vi "Loop_SM.vi"() -> ()   [LabVIEW 2017, in "Lift.lvlib"]
uses:
  Lift.lvlib
  CLUSTER_CMD_SM_Lift_Rotate.ctl
  ENUM_SM_Rotate_Positions.ctl
  _SHARE ALL/TypeDef Share All/CLUSTER_TalonInput.ctl
  System Drivers/Phoenix-LabVIEW/Motor Controller/Controls/CTRE_Phoenix_MotorControl_ControlMode.ctl
  TypeDef/CLUSTER_PID.ctl
  ENUM_SM_State.ctl
  CLUSTER_ACT_Lift Output.ctl
  _SHARE ALL/RoboRio Share All/SRX Share All/TypeDefs SRX/Cluster_SRX_General Data.ctl
  _SHARE ALL/RoboRio Share All/SRX Share All/TypeDefs SRX/Cluster_SRX_Common Runtime Data.ctl
  _SHARE ALL/RoboRio Share All/SRX Share All/TypeDefs SRX/Cluster_SRX_Error Calculations.ctl
  _SHARE ALL/RoboRio Share All/SRX Share All/TypeDefs SRX/Cluster_SRX_Voltage Out Data.ctl
  _SHARE ALL/RoboRio Share All/SRX Share All/TypeDefs SRX/Cluster_SRX_Sensor Out Data.ctl
  _SHARE ALL/RoboRio Share All/SRX Share All/TypeDefs SRX/Cluster_SRX_Sensor Quad Data.ctl
  _SHARE ALL/RoboRio Share All/SRX Share All/TypeDefs SRX/Cluster_SRX_Analog In Data.ctl
  _SHARE ALL/RoboRio Share All/SRX Share All/TypeDefs SRX/Cluster_SRX_PWM Sensor Data.ctl
  _SHARE ALL/RoboRio Share All/SRX Share All/TypeDefs SRX/Cluster_SRX_F and R Limit Indicators.ctl
  ENUM_SM_Action.ctl
  Globals/Global_Device_IDs.vi
  _SHARE ALL/Global Share All/Global_STOP.vi
  Global_CMD.vi
  Global_ACT Write_Data Out.vi
  Global_SM Write_Data Out.vi
panel:
  out "State":T1
  out "SM Output":T2 {"Talon Mode" items=["PercentOutput"=0, "Position"=1, "Velocity"=2, "Current"=3, "Follower"=5, "MotionProfile"=6, "MotionMagic"=7, "MotionMagicArc"=8, "MotionProfileArc"=10, "Disabled"=15]}
  out "SM CMD Input":T5={"Enable System"=TRUE, "Rotate Position"=enum."Neutral: 0", "Manual Velocity"=0.0, "Manual Mode"=FALSE}
  out "Cycle Time (S)":dbl format="%.3g"
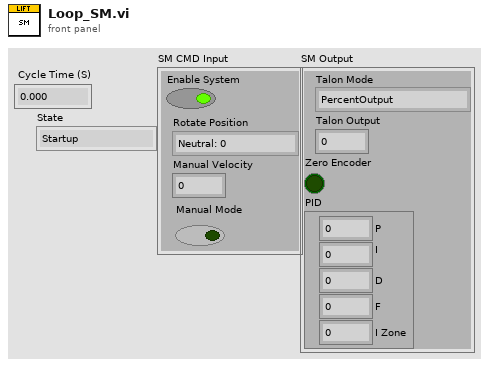
[diagram p1: front panel]
types:
  T1 = typedef "Lift.lvlib/ENUM_SM_State.ctl" = enum16{"Startup", "Idle", "Manual", "Position - Moving", "Position - Holding", "Shutdown"}
  T2 = typedef "CLUSTER_TalonInput.ctl" = cluster{"Talon Mode":T3, "Talon Output":dbl, "Zero Encoder":bool, "PID":T4}
  T3 = typedef "CTRE_Phoenix_MotorControl_ControlMode.ctl" = u16
  T4 = typedef "CLUSTER_PID.ctl" = cluster{"P":dbl, "I":dbl, "D":dbl, "F":dbl, "I Zone":dbl}
  T5 = typedef "Lift.lvlib/CLUSTER_CMD_SM_Lift_Rotate.ctl" = cluster{"Enable System":bool, "Rotate Position":T6, "Manual Velocity":dbl, "Manual Mode":bool}
  T6 = typedef "Lift.lvlib/ENUM_SM_Rotate_Positions.ctl" = enum16{"Neutral: 0", "Pickup: 0", "Exchange: 0", "Switch: 0", "Scale: 0", "Climb: 0"}
  T7 = typedef "Lift.lvlib/CLUSTER_ACT_Lift Output.ctl" = cluster{"Device Info Out":T8, "Common Runtime Data Out":T9, "Quad Sensor Data Out":T13, "Analog Sensor Data Out":T14, "PWM Data Out":T15, "Hard Limits Out":T16}
  T8 = typedef "Cluster_SRX_General Data.ctl" = cluster{"Device ID":i32, "Firmware Version":i32, "Inverted?":bool, "Has Reset Occurred?":bool}
  T9 = typedef "Cluster_SRX_Common Runtime Data.ctl" = cluster{"Calc":T10, "Voltage ":T11, "Sensor":T12, "Current":dbl, "Temp":dbl}
  T10 = typedef "Cluster_SRX_Error Calculations.ctl" = cluster{"Error":i32, "D-Error":dbl, "I-Acc":dbl}
  T11 = typedef "Cluster_SRX_Voltage Out Data.ctl" = cluster{"Percent":dbl, "Output":dbl, "Bus":dbl}
  T12 = typedef "Cluster_SRX_Sensor Out Data.ctl" = cluster{"Pos":i32, "Vel":i32}
  T13 = typedef "Cluster_SRX_Sensor Quad Data.ctl" = cluster{"Position":i32, "Velocity":i32, "Quad A Pin":bool, "Quad B Pin":bool, "Quad Idx Pin":bool}
  T14 = typedef "Cluster_SRX_Analog In Data.ctl" = cluster{"WithOv":i32, "Raw":i32, "Velocity":i32}
  T15 = typedef "Cluster_SRX_PWM Sensor Data.ctl" = cluster{"Position":i32, "Velocity":i32, "High(us)":i32, "Period(us)":i32}
  T16 = typedef "Cluster_SRX_F and R Limit Indicators.ctl" = cluster{"Forward Closed?":bool, "Reverse Closed?":bool}
  T17 = typedef "Lift.lvlib/ENUM_SM_Action.ctl" = enum16{"No Action", "Reset Time", "Reset All", "Reset Encoder", "Manual", "Position", "Set PID 1", "Disable Motor"}
  T18 = typedef "CLUSTER_Arm_Device_IDs.ctl" = cluster{"Master":T19, "Slave":T19}
  T19 = typedef "CLUSTER_Talon_Setup.ctl" = cluster{"Open Data":T20, "Current Config Data":T21, "Sensor Config":T22, "Hard Limits":T24, "Motion Magic Config Data":T26, "PIDF":T27, "Maximum Integral Accumulator Value":dbl, "AllowableClosedLoop":i32, "Limits":T28, "Output Config":T29}
  T20 = typedef "Cluster_SRX_OPEN Data.ctl" = cluster{"SRX ID":u8, "Invert Output":bool}
  T21 = typedef "Cluster_SRX_Current Config.ctl" = cluster{"Enable Current Limit?":bool, "Peak Current (Amps)":i32, "Peak Current Maximum Duration (ms)":i32, "Continuous Current Limit (Amps)":i32}
  T22 = typedef "Cluster_SRX_Sensor Config.ctl" = cluster{"Feedback Device":T23, "PhaseSensor":bool}
  T23 = typedef "CTRE_Phoenix_MotorControl_FeedbackDevice.ctl" = i8
  T24 = typedef "Cluster_SRX_Config Hard Limits.ctl" = cluster{"Fwd Enable":bool, "Rev Enable":bool, "Fwd NO-NC":T25, "Rev NO-NC":T25}
  T25 = typedef "CTRE_Phoenix_MotorControl_LimitSwitchNormal.ctl" = enum16{"Normally Open", "Normally Closed", "Disabled"}
  T26 = typedef "Cluster_SRX_Motion Magic Config Data.ctl" = cluster{"Cruise Velocity":i32, "Acceleration":i32}
  T27 = typedef "Cluster_SRX_PIDF.ctl" = cluster{"P":dbl, "I":dbl, "D":dbl, "F":dbl, "I Zone":dbl}
  T28 = typedef "Cluster_SRX_Config Soft Limits.ctl" = cluster{"Max":i32, "Min":i32, "Max Enable":bool, "Min Enable":bool}
  T29 = typedef "Cluster_SRX_Config Voltage Output.ctl" = cluster{"Invert?":bool, "Neutral Mode":T30, "Deadband (-1to1)":dbl, "Ramp Time Off to Full (S)":dbl, "Peak  (-1to1)":T31, "Nominal  (-1to1)":T31}
  T30 = typedef "CTRE_Phoenix_MotorControl_NeutralMode.ctl" = enum8{"EEPROMSetting", "Override to Coast", "Override to Brake"}
  T31 = typedef "Cluster_SRX_Forward and Reverse.ctl" = cluster{"Forward":dbl, "Reverse":dbl}
  T32 = cluster{"State":T1, "Previous State":T1, "Current Time":timestamp, "Previous Time":timestamp, "Start Time":timestamp, "Target Time (ms)":u32, "Cycle Time(S)":dbl, "Lift_Output":T7, "SM CMD Input":T5, "SM Output":T2, "Lift Setup":T18, "Manual Counter":i32}
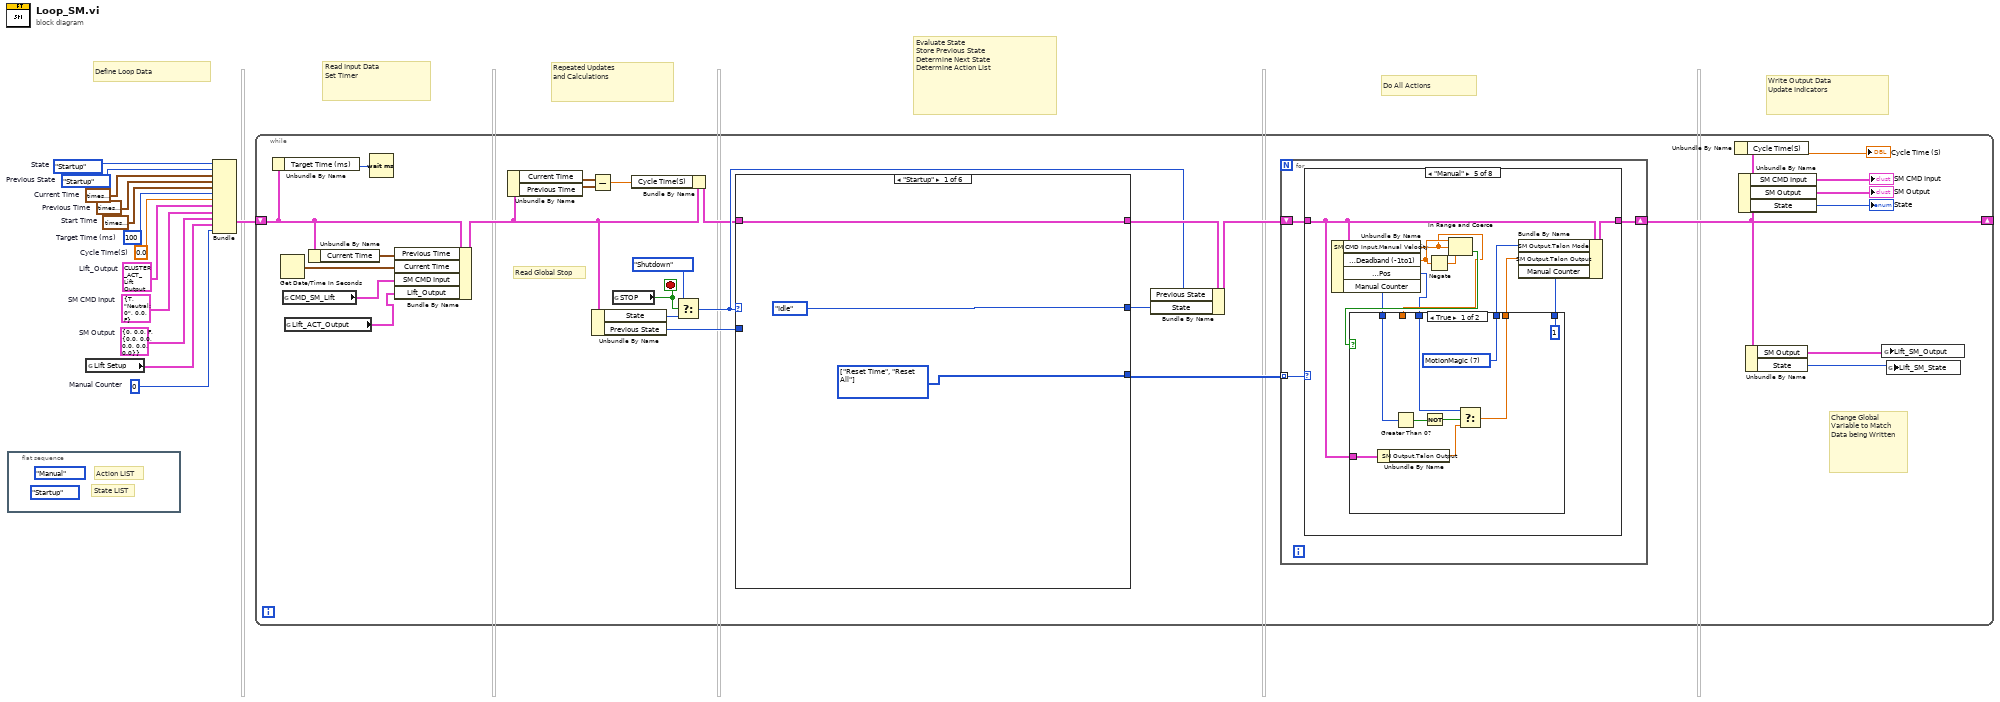
[diagram p0: block diagram]
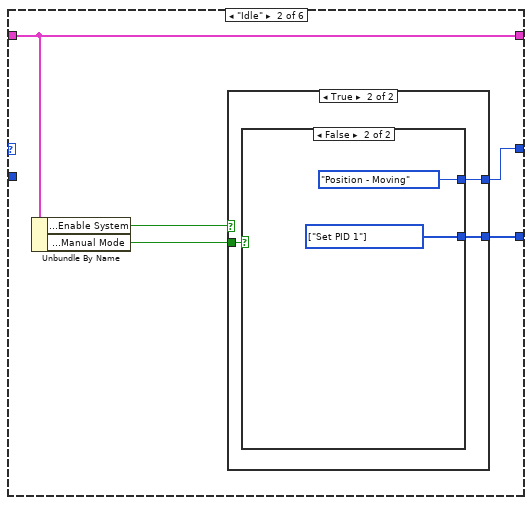
[diagram p2: hidden frame]
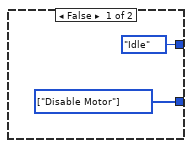
[diagram p3: hidden frame]
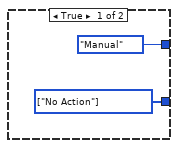
[diagram p4: hidden frame]
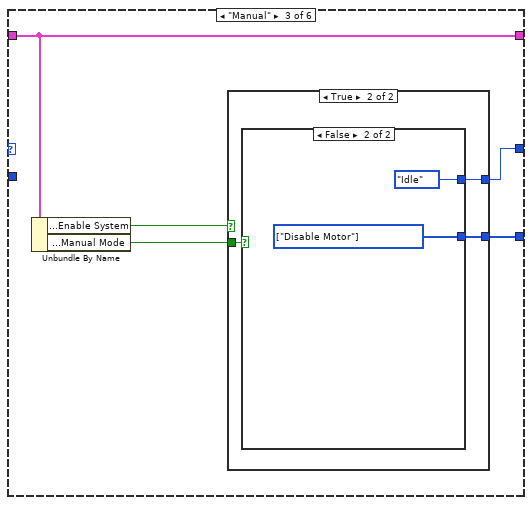
[diagram p5: hidden frame]
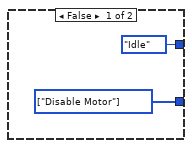
[diagram p6: hidden frame]
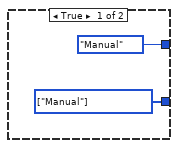
[diagram p7: hidden frame]
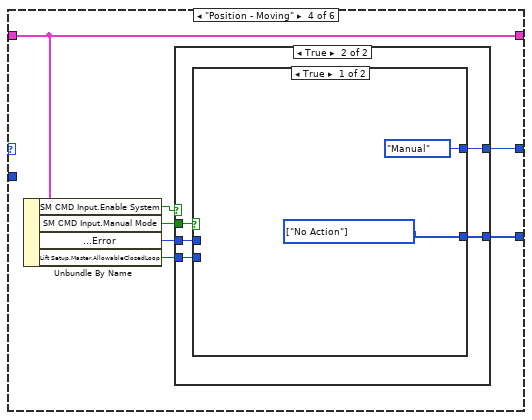
[diagram p8: hidden frame]
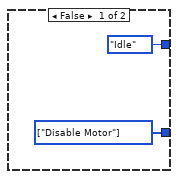
[diagram p9: hidden frame]
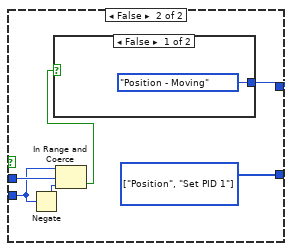
[diagram p10: hidden frame]
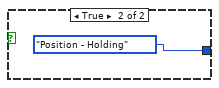
[diagram p11: hidden frame]
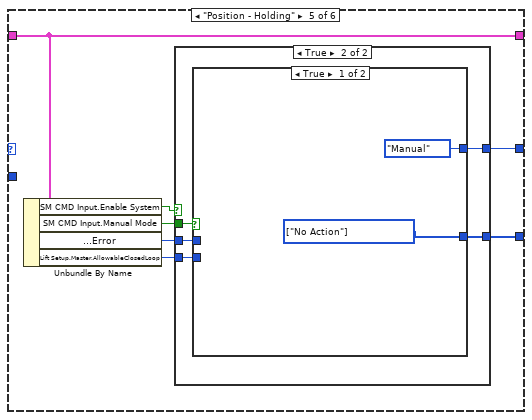
[diagram p12: hidden frame]
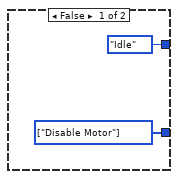
[diagram p13: hidden frame]
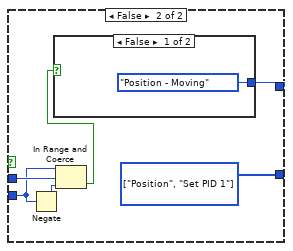
[diagram p14: hidden frame]
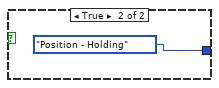
[diagram p15: hidden frame]
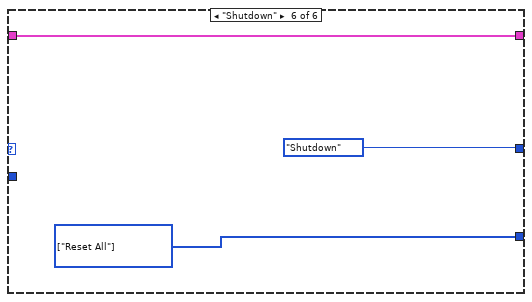
[diagram p16: hidden frame]
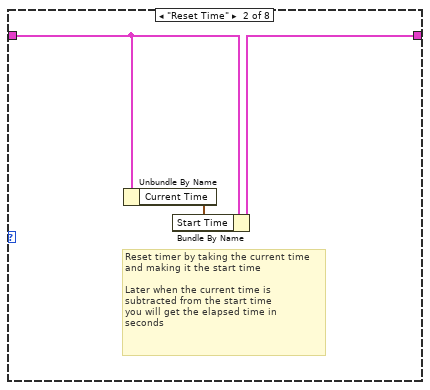
[diagram p18: hidden frame]
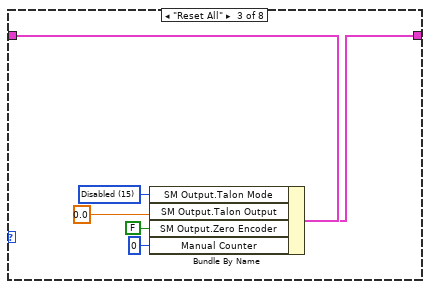
[diagram p19: hidden frame]
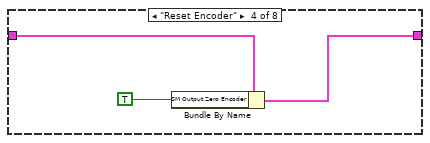
[diagram p20: hidden frame]
diagram:
  w1 = 0  # Manual Counter
  w3 = T2 {"Talon Mode"=0, "Talon Output"=0.0, "Zero Encoder"=FALSE, "PID"={"P"=0.0, "I"=0.0, "D"=0.0, "F"=0.0, "I Zone"=0.0}}  # SM Output
  w4 = T5 {"Enable System"=TRUE, "Rotate Position"=enum."Neutral: 0", "Manual Velocity"=0.0, "Manual Mode"=FALSE}  # SM CMD Input
  w5 = T7 {"Device Info Out"={"Device ID"=0, "Firmware Version"=0, "Inverted?"=FALSE, "Has Reset Occurred?"=FALSE}, "Common Runtime Data Out"={"Calc"={"Error"=0, "D-Error"=0.0, "I-Acc"=0.0}, "Voltage "={"Percent"=0.0, "Output"=0.0, "Bus"=0.0}, "Sensor"={"Pos"=0, "Vel"=0}, "Current"=0.0, "Temp"=0.0}, "Quad Sensor Data Out"={"Position"=0, "Velocity"=0, "Quad A Pin"=FALSE, "Quad B Pin"=FALSE, "Quad Idx Pin"=FALSE}, "Analog Sensor Data Out"={"WithOv"=0, "Raw"=0, "Velocity"=0}, "PWM Data Out"={"Position"=0, "Velocity"=0, "High(us)"=0, "Period(us)"=0}, "Hard Limits Out"={"Forward Closed?"=FALSE, "Reverse Closed?"=FALSE}}  # Lift_Output
  w6 = 0.0  # Cycle Time(S)
  w7 = ENUM_SM_State."Startup"  # Previous State
  w8 = timestamp(0 s since 1904-01-01)  # Previous Time
  w9 = u32 100  # Target Time (ms)
  w10 = timestamp(0 s since 1904-01-01)  # Start Time
  w11 = timestamp(0 s since 1904-01-01)  # Current Time
  w12 = ENUM_SM_State."Startup"  # State
  # "Define Loop Data"
  # "Repeated Updates\nand Calculations"
  # "Read Input Data\nSet Timer"
  # "Evaluate State\nStore Previous State\nDetermine Next State\nDetermine Action List"
  # "Do All Actions"
  # "Write Output Data\nUpdate Indicators"
  n1 = flat-sequence {
    frame #0 {
      (unwired) ENUM_SM_State."Startup" ("State")
      (unwired) ENUM_SM_Action."Manual" ("Action")
      # "State LIST"
      # "Action LIST"
    }
  }
  n2 = global read "Global_Device_IDs.vi" "Lift Setup"() -> (w2:T18)
  n3 = Bundle("State"=w12, "Previous State"=w7, "Current Time"=w11, "Previous Time"=w8, "Start Time"=w10, "Target Time (ms)"=w9, "Cycle Time(S)"=w6, "Lift_Output"=w5, "SM CMD Input"=w4, "SM Output"=w3, "Lift Setup"=w2, "Manual Counter"=w1) -> (w13:T32)  [unwired: 1 in]
  n4 = while {
    shift-right: [w29] -> _
    shift-left: w13 -> [w32]
    stop <- w37 stop-if-true
    # "Change Global\nVariable to Match\nData being Written"
    # "Read Global Stop"
    n5 = Unbundle By Name(w32) -> ("Target Time (ms)"=w34:u32)
    n6 = Get Date/Time In Seconds() -> (seconds since 1Jan1904=w40:timestamp)
    n7 = global read "Global_CMD.vi" "CMD_SM_Lift"() -> (w21:T5)
    n8 = global read "Global_ACT Write_Data Out.vi" "Lift_ACT_Output"() -> (w20:T7)
    n9 = Unbundle By Name(w32) -> ("Current Time"=w33:timestamp)
    n10 = Wait (ms)(milliseconds to wait=w34) -> ()  [unwired: 1 out]
    n11 = Bundle By Name(cluster=w32, "Previous Time"=w33, "Current Time"=w40, "SM CMD Input"=w21, "Lift_Output"=w20) -> (w25:T32)
    n12 = Unbundle By Name(w25) -> ("Current Time"=w26:timestamp, "Previous Time"=w27:timestamp)
    n13 = Subtract(x=w26, y=w27) -> (x-y=w23:dbl)
    n14 = Unbundle By Name(w25) -> ("State"=w35:T1, "Previous State"=w31:T1)
    n15 = global read "Global_STOP.vi" "STOP"() -> (w37:bool)
    n16 = Bundle By Name(cluster=w25, "Cycle Time(S)"=w23) -> (w24:T32)
    n17 = Select(t=ENUM_SM_State."Shutdown" ("State"), s=w37, f=w35) -> (s? t:f=w30:T1)
    n18 = case shown="\"Startup\"" w30 {
      tunnel: w24 -> [w43 w48 w62 w78 w102 w122]
      tunnel: [w43 w48 w62 w78 w102 w122] -> w38
      tunnel: [w42 w44 w58 w74 w98 w121] -> w22
      tunnel: w31 -> [_ _ _ _ _ _]
      tunnel: [ENUM_SM_State."Idle" ("State") w45 w59 w73 w97 ENUM_SM_State."Shutdown" ("State")] -> w19
      frame "Startup" {
        w42 = T17[] [enum."Reset Time", enum."Reset All"] items=["No Action", "Reset Time", "Reset All", "Reset Encoder", "Manual", "Position", "Set PID 1", "Disable Motor"] ("Actions")
      }
      frame "Idle" {
        n19 = Unbundle By Name(w48) -> ("SM CMD Input.Enable System"=w47:bool, "SM CMD Input.Manual Mode"=w46:bool)
        n20 = case shown="True" w47 {
          tunnel: w46 -> [_ w53]
          tunnel: [ENUM_SM_State."Idle" ("State") w52] -> w45
          tunnel: [w49 w51] -> w44
          frame False {
            w49 = T17[] [enum."Disable Motor"] items=["No Action", "Reset Time", "Reset All", "Reset Encoder", "Manual", "Position", "Set PID 1", "Disable Motor"] ("Actions")
          }
          frame True {
            n21 = case shown="False" w53 {
              tunnel: [ENUM_SM_State."Manual" ("State") ENUM_SM_State."Position - Moving" ("State")] -> w52
              tunnel: [w54 w56] -> w51
              frame True {
                w54 = T17[] [enum."No Action"] items=["No Action", "Reset Time", "Reset All", "Reset Encoder", "Manual", "Position", "Set PID 1", "Disable Motor"] ("Actions")
              }
              frame False {
                w56 = T17[] [enum."Set PID 1"] items=["No Action", "Reset Time", "Reset All", "Reset Encoder", "Manual", "Position", "Set PID 1", "Disable Motor"] ("Actions")
              }
            }
          }
        }
      }
      frame "Manual" {
        n22 = Unbundle By Name(w62) -> ("SM CMD Input.Enable System"=w61:bool, "SM CMD Input.Manual Mode"=w60:bool)
        n23 = case shown="True" w61 {
          tunnel: w60 -> [_ w67]
          tunnel: [ENUM_SM_State."Idle" ("State") w66] -> w59
          tunnel: [w63 w65] -> w58
          frame False {
            w63 = T17[] [enum."Disable Motor"] items=["No Action", "Reset Time", "Reset All", "Reset Encoder", "Manual", "Position", "Set PID 1", "Disable Motor"] ("Actions")
          }
          frame True {
            n24 = case shown="False" w67 {
              tunnel: [ENUM_SM_State."Manual" ("State") ENUM_SM_State."Idle" ("State")] -> w66
              tunnel: [w68 w70] -> w65
              frame True {
                w68 = T17[] [enum."Manual"] items=["No Action", "Reset Time", "Reset All", "Reset Encoder", "Manual", "Position", "Set PID 1", "Disable Motor"] ("Actions")
              }
              frame False {
                w70 = T17[] [enum."Disable Motor"] items=["No Action", "Reset Time", "Reset All", "Reset Encoder", "Manual", "Position", "Set PID 1", "Disable Motor"] ("Actions")
              }
            }
          }
        }
      }
      frame "Position - Moving" {
        n25 = Unbundle By Name(w78) -> ("SM CMD Input.Enable System"=w72:bool, "SM CMD Input.Manual Mode"=w77:bool, "Lift_Output.Common Runtime Data Out.Calc.Error"=w76:i32, "Lift Setup.Master.AllowableClosedLoop"=w75:i32)
        n26 = case shown="True" w72 {
          tunnel: w77 -> [_ w85]
          tunnel: w76 -> [_ w84]
          tunnel: w75 -> [_ w83]
          tunnel: [w79 w82] -> w74
          tunnel: [ENUM_SM_State."Idle" ("State") w81] -> w73
          frame False {
            w79 = T17[] [enum."Disable Motor"] items=["No Action", "Reset Time", "Reset All", "Reset Encoder", "Manual", "Position", "Set PID 1", "Disable Motor"] ("Actions")
          }
          frame True {
            n27 = case shown="True" w85 {
              tunnel: w84 -> [_ w93]
              tunnel: w83 -> [_ w92]
              tunnel: [w86 w89] -> w82
              tunnel: [ENUM_SM_State."Manual" ("State") w88] -> w81
              frame True {
                w86 = T17[] [enum."No Action"] items=["No Action", "Reset Time", "Reset All", "Reset Encoder", "Manual", "Position", "Set PID 1", "Disable Motor"] ("Actions")
              }
              frame False {
                w89 = T17[] [enum."Position", enum."Set PID 1"] items=["No Action", "Reset Time", "Reset All", "Reset Encoder", "Manual", "Position", "Set PID 1", "Disable Motor"] ("Actions")
                n28 = Negate(x=w92) -> (-x=w91:i32)
                n29 = In Range and Coerce(upper limit=w92, x=w93, lower limit=w91) -> (In Range?=w90:bool)  [unwired: 1 out]
                n30 = case shown="False" w90 {
                  tunnel: [ENUM_SM_State."Position - Moving" ("State") ENUM_SM_State."Position - Holding" ("State")] -> w88
                  frame False {
                  }
                  frame True {
                  }
                }
              }
            }
          }
        }
      }
      frame "Position - Holding" {
        n31 = Unbundle By Name(w102) -> ("SM CMD Input.Enable System"=w96:bool, "SM CMD Input.Manual Mode"=w101:bool, "Lift_Output.Common Runtime Data Out.Calc.Error"=w100:i32, "Lift Setup.Master.AllowableClosedLoop"=w99:i32)
        n32 = case shown="True" w96 {
          tunnel: w101 -> [_ w109]
          tunnel: w100 -> [_ w108]
          tunnel: w99 -> [_ w107]
          tunnel: [w103 w106] -> w98
          tunnel: [ENUM_SM_State."Idle" ("State") w105] -> w97
          frame False {
            w103 = T17[] [enum."Disable Motor"] items=["No Action", "Reset Time", "Reset All", "Reset Encoder", "Manual", "Position", "Set PID 1", "Disable Motor"] ("Actions")
          }
          frame True {
            n33 = case shown="True" w109 {
              tunnel: w108 -> [_ w117]
              tunnel: w107 -> [_ w116]
              tunnel: [w110 w113] -> w106
              tunnel: [ENUM_SM_State."Manual" ("State") w112] -> w105
              frame True {
                w110 = T17[] [enum."No Action"] items=["No Action", "Reset Time", "Reset All", "Reset Encoder", "Manual", "Position", "Set PID 1", "Disable Motor"] ("Actions")
              }
              frame False {
                w113 = T17[] [enum."Position", enum."Set PID 1"] items=["No Action", "Reset Time", "Reset All", "Reset Encoder", "Manual", "Position", "Set PID 1", "Disable Motor"] ("Actions")
                n34 = Negate(x=w116) -> (-x=w115:i32)
                n35 = In Range and Coerce(upper limit=w116, x=w117, lower limit=w115) -> (In Range?=w114:bool)  [unwired: 1 out]
                n36 = case shown="False" w114 {
                  tunnel: [ENUM_SM_State."Position - Moving" ("State") ENUM_SM_State."Position - Holding" ("State")] -> w112
                  frame False {
                  }
                  frame True {
                  }
                }
              }
            }
          }
        }
      }
      frame "Shutdown" {
        w121 = T17[] [enum."Reset All"] items=["No Action", "Reset Time", "Reset All", "Reset Encoder", "Manual", "Position", "Set PID 1", "Disable Motor"] ("Actions")
      }
    }
    n37 = Bundle By Name(cluster=w38, "Previous State"=w30, "State"=w19) -> (w39:T32)
    n38 = for {
      tunnel: w22 -> [w125] mode=indexing
      shift-right: [w124] -> w29
      shift-left: w39 -> [w123]
      n39 = case shown="\"Manual\"" w125 {
        tunnel: w123 -> [w126 w129 w135 w138 w139 w169 w172 w176]
        tunnel: [w126 w128 w134 w137 w146 w170 w173 w175] -> w124
        frame "No Action" {
        }
        frame "Reset Time" {
          # "Reset timer by taking the current time\nand making it the start time\n\nLater when the current time is \nsubtracted from the start time\nyou will get the elapsed time in \nseconds"
          n40 = Unbundle By Name(w129) -> ("Current Time"=w127:timestamp)
          n41 = Bundle By Name(cluster=w129, "Start Time"=w127) -> (w128:T32)
        }
        frame "Reset All" {
          w133 = T3 15 items=["PercentOutput"=0, "Position"=1, "Velocity"=2, "Current"=3, "Follower"=5, "MotionProfile"=6, "MotionMagic"=7, "MotionMagicArc"=8, "MotionProfileArc"=10, "Disabled"=15] ("SM Output.Talon Mode")
          n42 = Bundle By Name(cluster=w135, "SM Output.Talon Mode"=w133, "SM Output.Talon Output"=0.0, "SM Output.Zero Encoder"=FALSE, "Manual Counter"=0) -> (w134:T32)
        }
        frame "Reset Encoder" {
          n43 = Bundle By Name(cluster=w138, "SM Output.Zero Encoder"=TRUE) -> (w137:T32)
        }
        frame "Manual" {
          n44 = Unbundle By Name(w139) -> ("SM CMD Input.Manual Velocity"=w145:dbl, "Lift Setup.Master.Output Config.Deadband (-1to1)"=w149:dbl, "Lift_Output.Common Runtime Data Out.Sensor.Pos"=w141:i32, "Manual Counter"=w140:i32)
          n45 = Negate(x=w149) -> (-x=w148:dbl)
          n46 = In Range and Coerce(upper limit=w149, x=w145, lower limit=w148) -> (In Range?=w147:bool)  [unwired: 1 out]
          n47 = case shown="True" w147 {
            tunnel: w145 -> [_ w160]
            tunnel: [w158 w161] -> w144
            tunnel: [w150 w160] -> w143
            tunnel: [1 0] -> w142
            tunnel: w141 -> [w156 _]
            tunnel: w140 -> [w153 _]
            tunnel: w139 -> [w152 _]
            frame True {
              w158 = T3 7 items=["PercentOutput"=0, "Position"=1, "Velocity"=2, "Current"=3, "Follower"=5, "MotionProfile"=6, "MotionMagic"=7, "MotionMagicArc"=8, "MotionProfileArc"=10, "Disabled"=15] ("SM Output.Talon Mode")
              n48 = Unbundle By Name(w152) -> ("SM Output.Talon Output"=w151:dbl)
              n49 = Greater Than 0?(x=w153) -> (x > 0?=w154:bool)
              n50 = Not(x=w154) -> (.not. x?=w155:bool)
              n51 = Select(t=w156, s=w155, f=w151) -> (s? t:f=w150:dbl)
            }
            frame False {
              w161 = T3 0 items=["PercentOutput"=0, "Position"=1, "Velocity"=2, "Current"=3, "Follower"=5, "MotionProfile"=6, "MotionMagic"=7, "MotionMagicArc"=8, "MotionProfileArc"=10, "Disabled"=15] ("SM Output.Talon Mode")
            }
          }
          n52 = Bundle By Name(cluster=w139, "SM Output.Talon Mode"=w144, "SM Output.Talon Output"=w143, "Manual Counter"=w142) -> (w146:T32)
        }
        frame "Position" {
          n53 = Unbundle By Name(w169) -> ("SM CMD Input.Rotate Position"=w163:T6)
          n54 = Format Into String(w163) -> (resulting string=w168:string)  [unwired: 3 in, 1 out]
          n55 = Match Pattern(string=w168, regular expression=":") -> (before substring=w166:string, after substring=w165:string)  [unwired: 1 in, 2 out]
          n56 = call <vilib>:"Trim Whitespace.vi"("string"=w166) -> ()  [unwired: 1 in, 1 out]
          n57 = call <vilib>:"Trim Whitespace.vi"("string"=w165) -> ("trimmed string"=w164:string)  [unwired: 1 in]
          n58 = Decimal String To Number(string=w164) -> (number=w162:i32)  [unwired: 2 in, 1 out]
          n59 = Bundle By Name(cluster=w169, "SM Output.Talon Output"=w162) -> (w170:T32)
        }
        frame "Set PID 1" {
          n60 = Unbundle By Name(w172) -> ("Lift Setup.Master.PIDF"=w171:T27)
          n61 = Bundle By Name(cluster=w172, "SM Output.PID"=w171) -> (w173:T32)
        }
        frame "Disable Motor" {
          w174 = T3 15 items=["PercentOutput"=0, "Position"=1, "Velocity"=2, "Current"=3, "Follower"=5, "MotionProfile"=6, "MotionMagic"=7, "MotionMagicArc"=8, "MotionProfileArc"=10, "Disabled"=15] ("SM Output.Talon Mode")
          n62 = Bundle By Name(cluster=w176, "SM Output.Talon Mode"=w174) -> (w175:T32)
        }
      }
    }
    n63 = Unbundle By Name(w29) -> ("Cycle Time(S)"=→"Cycle Time (S)":dbl)
    n64 = Unbundle By Name(w29) -> ("SM CMD Input"=→"SM CMD Input":T5, "SM Output"=→"SM Output":T2, "State"=→"State":T1)
    n65 = Unbundle By Name(w29) -> ("SM Output"=w17:T2, "State"=w18:T1)
    n66 = global write "Global_SM Write_Data Out.vi" "Lift_SM_Output"(w17) -> ()
    n67 = global write "Global_SM Write_Data Out.vi" "Lift_SM_State"(w18) -> ()
  }
